vi "PollEngine.Initialize.vi"(8 "error in (no error)":errorcluster, 9 "Parent VI":refnum<vi>, 10 "Parameters in":T3 {"Settings"."Data Refs"."Write Refs" format="%.0x"; "Settings"."Data Refs"."Read Refs" format="%.0x"; "Settings"."Write Locations"."DataType" items=["Boolean"=1, "SByte"=2, "Byte"=3, "Int16"=4, "UInt16"=5, "Int32"=6, "UInt32"=7, "Int64"=8, "UInt64"=9, "Float"=10, "Double"=11, "String"=12, "DateTime"=13, "ByteString"=15, "Array of Boolean"=101, "Array of SByte"=102, "Array of Byte"=103, "Array of Int16"=104, "Array of UInt16"=105, "Array of Int32"=106, "Array of UInt32"=107, "Array of Int64"=108, "Array of UInt64"=109, "Array of Float"=110, "Array of Double"=111, "Array of String"=112, "Array of DateTime"=113, "Array of ByteString"=115]; "Settings"."StatusRefs"."Chan Refs" format="%.0x"}, 11 "Parent":string) -> (0 "error out":errorcluster, 1 "notification":bool, 2 "Parameters out":T3 {"Settings"."Data Refs"."Write Refs" format="%.0x"; "Settings"."Data Refs"."Read Refs" format="%.0x"; "Settings"."Write Locations"."DataType" items=["Boolean"=1, "SByte"=2, "Byte"=3, "Int16"=4, "UInt16"=5, "Int32"=6, "UInt32"=7, "Int64"=8, "UInt64"=9, "Float"=10, "Double"=11, "String"=12, "DateTime"=13, "ByteString"=15, "Array of Boolean"=101, "Array of SByte"=102, "Array of Byte"=103, "Array of Int16"=104, "Array of UInt16"=105, "Array of Int32"=106, "Array of UInt32"=107, "Array of Int64"=108, "Array of UInt64"=109, "Array of Float"=110, "Array of Double"=111, "Array of String"=112, "Array of DateTime"=113, "Array of ByteString"=115]; "Settings"."StatusRefs"."Chan Refs" format="%.0x"}, 3 "Settings":T1)   [LabVIEW 2013, in "OPC UA Client Engine.lvlib"]
uses:
  OPC UA Client Engine.lvlib
  Types/PollEngine.Parameters.ctl
  Shared/Compiled.Settings.ctl
  Shared/Connection.Properties.ctl
  Shared/PollEngine.Settings.ctl
  <vilib>/NI Veristand/Custom Device API/Data Reference.ctl
  Shared/WriteData.Info.ctl
  Shared/ReadWriteRefs.ctl
  Types/PollEngine.StateVariables.ctl
  Stop FG/Stop Global Ref.ctl
  <vilib>/OPCUA/NI OPC UA Client.lvlib
  Stop FG/Stop FG.lvlib
  Inline Async API/Inline Async API.lvlib
  Error Handling API/Error Handling API.lvlib
  <vilib>/NI Veristand/Custom Device API/Custom Device API.lvlib
  Shared/OPC UA Client Shared.lvlib
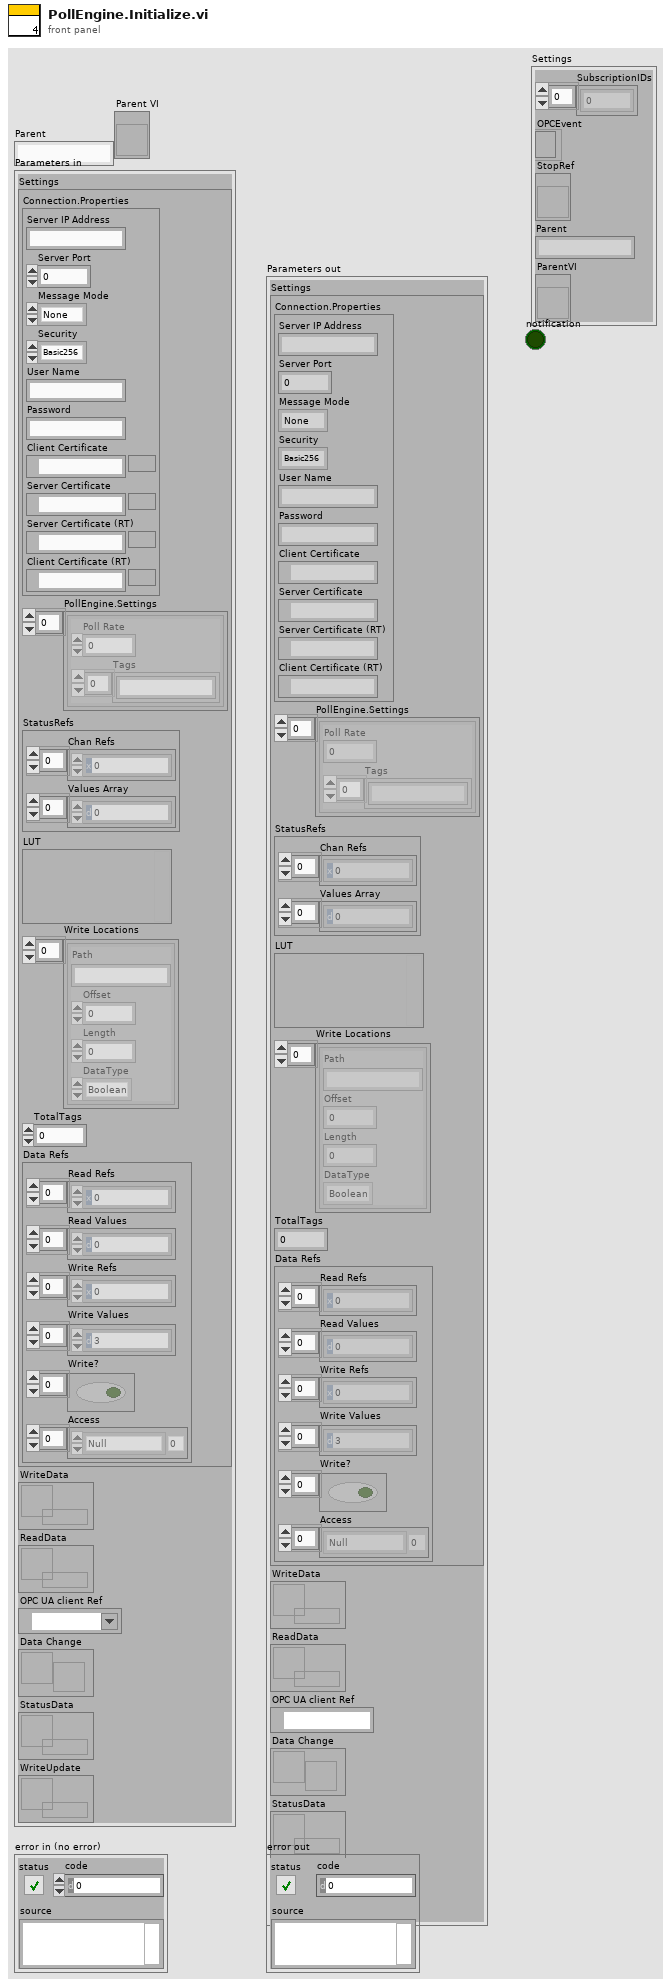
[diagram p1: front panel]
types:
  T1 = typedef "OPC UA Client Engine.lvlib/PollEngine.StateVariables.ctl" = cluster{"SubscriptionIDs":u32[], "OPCEvent":refnum<event-registration>, "StopRef":T2, "Parent":string, "ParentVI":refnum<vi>}
  T2 = typedef "OPC UA Client Engine.lvlib/Stop FG.lvlib/Stop Global Ref.ctl" = refnum<vi>
  T3 = typedef "OPC UA Client Engine.lvlib/PollEngine.Parameters.ctl" = cluster{"Settings":T4, "WriteData":refnum<k33>, "ReadData":refnum<k33>, "OPC UA client Ref":refnum<k21>, "Data Change":refnum<user-event>, "StatusData":refnum<k33>, "WriteUpdate":refnum<k33>}
  T4 = typedef "OPC UA Client Shared.lvlib/Compiled.Settings.ctl" = cluster{"Connection.Properties":T5, "PollEngine.Settings":T6[], "StatusRefs":cluster{"Chan Refs":T7[], "Values Array":dbl[]}, "LUT":variant, "Write Locations":T8[], "TotalTags":u32, "Data Refs":T9}
  T5 = typedef "OPC UA Client Shared.lvlib/Connection.Properties.ctl" = cluster{"Server IP Address":string, "Server Port":u16, "Message Mode":enum16{"None", "Sign", "Sign and Encrypt"}, "Security":enum16{"Basic256", "Basic128Rsa15"}, "User Name":string, "Password":string, "Client Certificate":path, "Server Certificate":path, "Server Certificate (RT)":path, "Client Certificate (RT)":path}
  T6 = typedef "OPC UA Client Shared.lvlib/PollEngine.Settings.ctl" = cluster{"Poll Rate":dbl, "Tags":string[]}
  T7 = typedef "Custom Device API.lvlib/Data Reference.ctl" = i32
  T8 = typedef "OPC UA Client Shared.lvlib/WriteData.Info.ctl" = cluster{"Path":string, "Offset":i32, "Length":i32, "DataType":u32}
  T9 = typedef "OPC UA Client Shared.lvlib/ReadWriteRefs.ctl" = cluster{"Read Refs":T7[], "Read Values":dbl[], "Write Refs":T7[], "Write Values":dbl[], "Write?":bool[], "Access":enum8{"Null", "Read", "Write", "Read&Write"}[]}
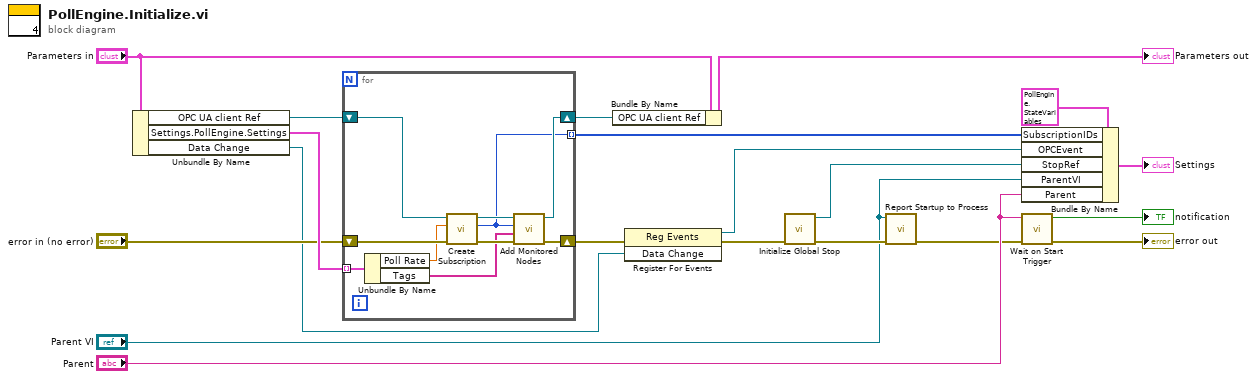
[diagram p0: block diagram]
diagram:
  n1 = Unbundle By Name("Parameters in") -> ("OPC UA client Ref"=w14:refnum<k21>, "Settings.PollEngine.Settings"=w15:T6[], "Data Change"=w5:refnum<user-event>)
  n2 = for {
    tunnel: [w26] -> w11 mode=indexing
    tunnel: w15 -> [w23] mode=indexing
    shift-right: [w27] -> w13
    shift-left: "error in (no error)" -> [w24]
    shift-right: [w28] -> w18
    shift-left: w14 -> [w25]
    n3 = Unbundle By Name(w23) -> ("Poll Rate"=w22:dbl, "Tags"=w21:string[])
    n4 = call <vilib>:"Create Subscription.vi"("error in (no error)"=w24, "update rate (1000 ms)"=w22, "OPC UA client refnum in"=w25) -> ("error out"=w29:errorcluster, "subscription ID out"=w26:u32, "OPC UA client refnum out"=w30:refnum<k21>)  [unwired: 6 in]
    n5 = call <vilib>:"Add Monitored Nodes.vi"("error in (no error)"=w29, "array of node path"=w21, "subscription ID in"=w26, "OPC UA client refnum in"=w30) -> ("error out"=w27:errorcluster, "OPC UA client refnum out"=w28:refnum<k21>)  [unwired: 5 in, 1 out]
  }
  n6 = Bundle By Name(cluster="Parameters in", "OPC UA client Ref"=w18) -> (→"Parameters out":T3)
  n7 = register-events(error in=w13, w5) -> (reference out=w8:refnum<event-registration>, error out=w16:errorcluster)  [unwired: 1 in]
  n8 = call "Initialize Global Stop.vi"("error in (no error)"=w16) -> ("error out"=w3:errorcluster, "vi reference"=w9:T2)  [unwired: 9 in]
  n9 = call "Report Startup to Process.vi"("Error"=w3, "This VI"="Parent VI") -> ("error out"=w2:errorcluster)  [unwired: 9 in]
  n10 = Bundle By Name(cluster=T1 {"SubscriptionIDs"=[], "OPCEvent"=refnum, "StopRef"=refnum, "Parent"="", "ParentVI"=refnum} ("output cluster"), "SubscriptionIDs"=w11, "OPCEvent"=w8, "StopRef"=w9, "ParentVI"="Parent VI", "Parent"="Parent") -> (→"Settings":T1)
  n11 = call "Wait on Start Trigger.vi"("error in (no error)"=w2, "Name"="Parent") -> ("error out"=→"error out":errorcluster, "notification"=→"notification":bool)  [unwired: 8 in]
